vi "Teleop.vi"(10 "Match Info":T2={"Autonomous Elapsed Seconds"=0.0, "TeleOp Elapsed Seconds"=0.0, "Disabled Elapsed Seconds"=0.0, "Visited Autonomous"=FALSE, "Visited TeleOp"=FALSE, "Visited Disabled"=FALSE, "Autonomous Settings"={"Autonomous Style"=enum."Independent", "VI Refnum"=refnum}}, 11 "Call Context":T3) -> ()   [LabVIEW 2017]
doc: "This VI is called for each TeleOp packet received from the DS where the robot is not disabled. It is often used to read from the joysticks and update I/O or to update setpoints for timed control loops. It should complete and return within 20 milliseconds or it may miss DS packets."
uses:
  <vilib>/Rock Robotics/WPI/DriverStation/WPI_DriverStationDerivedRobotMode.ctl
  <vilib>/Rock Robotics/WPI/DriverStation/WPI_DriverStationMatch Info.ctl
  Type Definitions/Teleop States.ctl
  Type Definitions/Joystick Axes.ctl
  Type Definitions/joystick Buttons.ctl
  <vilib>/Rock Robotics/WPI/ThirdParty/Phoenix-LabVIEW/Motor Controller/Controls/CTRE_Phoenix_MotorControl_ControlMode.ctl
  <vilib>/Rock Robotics/WPI/Utilities/WPI_GetSetVariantRefNum.vi
  <vilib>/Rock Robotics/Network Tables/NT Write Number.vi
panel:
  in  "Manual Control":bool
  in  "Right Slide":dbl(slide) min=-0.15 max=0.15 step=0.01 scale=-0.2..0.2 scale format="%.2f"
  in  "Left Slide":dbl(slide) min=-0.15 max=0.15 step=0.01 scale=-0.2..0.2 scale format="%.2f"
  in  "Teleop Analyctical Data":T1
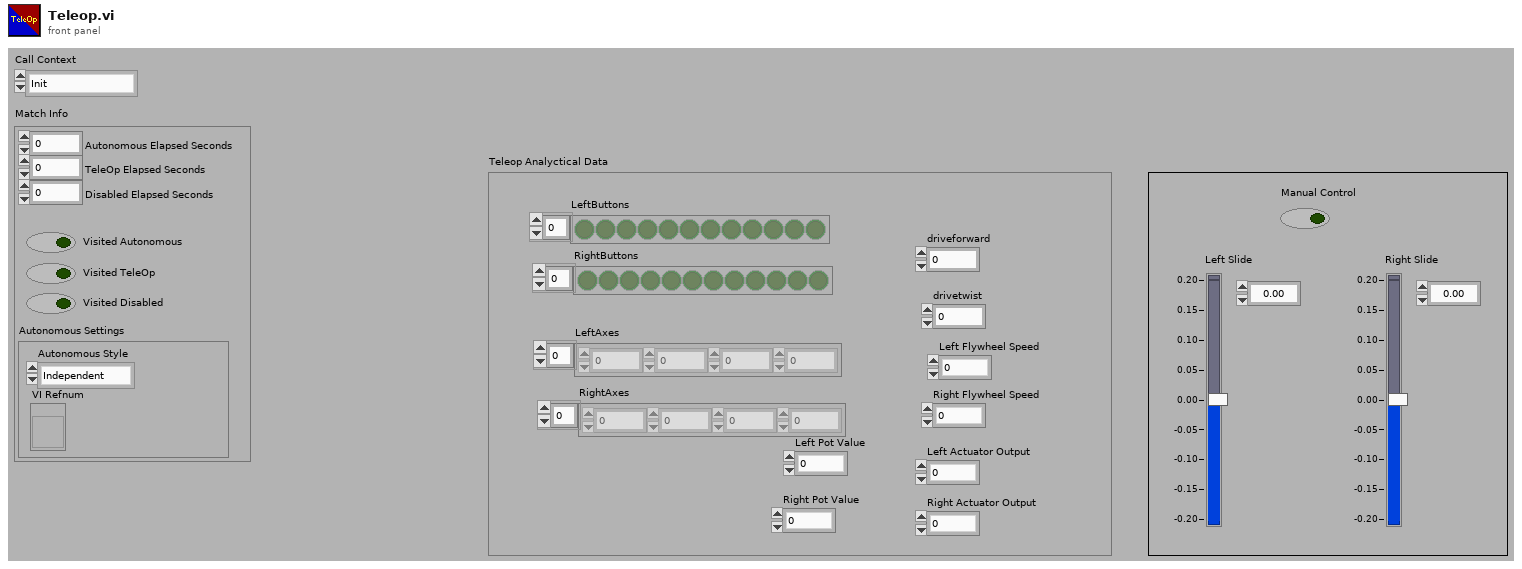
[diagram p1: front panel]
types:
  T1 = cluster{"LeftButtons":bool[], "RightButtons":bool[], "LeftAxes":dbl[], "RightAxes":dbl[], "driveforward":dbl, "drivetwist":dbl, "Left Flywheel Speed":dbl, "Right Flywheel Speed":dbl, "Left Actuator Output":dbl, "Right Actuator Output":dbl, "Left Pot Value":dbl, "Right Pot Value":dbl}
  T2 = typedef "WPI_DriverStationMatch Info.ctl" = cluster{"Autonomous Elapsed Seconds":dbl, "TeleOp Elapsed Seconds":dbl, "Disabled Elapsed Seconds":dbl, "Visited Autonomous":bool, "Visited TeleOp":bool, "Visited Disabled":bool, "Autonomous Settings":cluster{"Autonomous Style":enum16{"Iterative", "Independent"}, "VI Refnum":refnum<vi>}}
  T3 = typedef "WPI_DriverStationDerivedRobotMode.ctl" = enum16{"Init", "Execute", "Stop"}
  T4 = typedef "Teleop States.ctl" = enum16{"Start", "i_leftJoystick", "i_RightJoystick", "i_pot", "c_drive", "c_actuator", "c_flywheels", "output", "output actuator", "End"}
  T5 = typedef "Joystick Axes.ctl" = enum16{"X Axis", "Y Axis", "Twist", "Throttle"}
  T6 = typedef "joystick Buttons.ctl" = enum16{"Trigger", "Thumb", "buttom2", "buttom3", "button4", "button5", "button6"}
  T7 = typedef "WPI_JoystickDevRef.ctl" = cluster{"Device":T8}
  T8 = typedef "WPI_JoystickDeviceEnum.ctl" = enum16{"USB 0", "USB 1", "USB 2", "USB 3", "USB 4", "USB 5"}
  T9 = typedef "WPI_PotentiometerDevRef.ctl" = cluster{"DevStatus":errorcluster, "Analog Channel":T10, "Invert Output":bool}
  T10 = typedef "FPGA_AIChannel.ctl" = enum8{"AI 0", "AI 1", "AI 2", "AI 3", "AI MXP 0", "AI MXP 1", "AI MXP 2", "AI MXP 3", "Invalid"}
  T11 = typedef "CTRE_Phoenix_MotorControl_ControlMode.ctl" = u16
  T12 = typedef "WPI_RobotDriveDevRef.ctl" = cluster{"DevStatus":errorcluster, "Motors[]":T13[], "Square Inputs":bool, "Max Output":dbl}
  T13 = typedef "WPI_MotorControlDeviceRef.ctl" = cluster{"DeviceStatus":errorcluster, "Type":T14, "PWM":cluster{"PWM Channel":T15, "DeadBand":T16}, "CAN":cluster{"Device Number":u8, "SetOutput VI Ref":variant, "GetOutput VI Ref":variant, "Enable VI Ref":variant, "Disable VI Ref":variant, "Data":variant}, "Invert":bool, "DIO PWM":cluster{"PWM \"Enable\" Channel":T15, "DIOChannel":T17, "PWM Rate":dbl}}
  T14 = typedef "WPI_MotorControlType.ctl" = enum16{"PWM", "CAN", "DIO PWM"}
  T15 = typedef "FPGA_DIOPWMChannel.ctl" = enum8{"PWM 0", "PWM 1", "PWM 2", "PWM 3", "PWM 4", "PWM 5", "PWM 6", "PWM 7", "PWM 8", "PWM 9", "PWM MXP 0", "PWM MXP 1", "PWM MXP 2", "PWM MXP 3", "PWM MXP 4", "PWM MXP 5", "PWM MXP 6", "PWM MXP 7", "PWM MXP 8", "PWM MXP 9", "Invalid"}
  T16 = typedef "WPI_PWMDeadband.ctl" = cluster{"Name":string, "maxPositivePwm":i32, "minPositivePwm":i32, "centerPwm":i32, "maxNegativePwm":i32, "minNegativePwm":i32, "angularRange":u16}
  T17 = typedef "FPGA_DIOChannel.ctl" = enum8{"DIO 0", "DIO 1", "DIO 2", "DIO 3", "DIO 4", "DIO 5", "DIO 6", "DIO 7", "DIO 8", "DIO 9", "DIO MXP 0", "DIO MXP 1", "DIO MXP 2", "DIO MXP 3", "DIO MXP 4", "DIO MXP 5", "DIO MXP 6", "DIO MXP 7", "DIO MXP 8", "DIO MXP 9", "DIO MXP 10", "DIO MXP 11", "DIO MXP 12", "DIO MXP 13", "DIO MXP 14", "DIO MXP 15", "SPI Port CS1", "SPI Port CS2", "SPI Port CS3", "SPI Port MISO", "SPI Port MOSI", "Invalid"}
  T18 = typedef "WPI_ServoDeviceRef.ctl" = cluster{"DeviceStatus":errorcluster, "PWM Channel":T15, "DeadBand":T16}
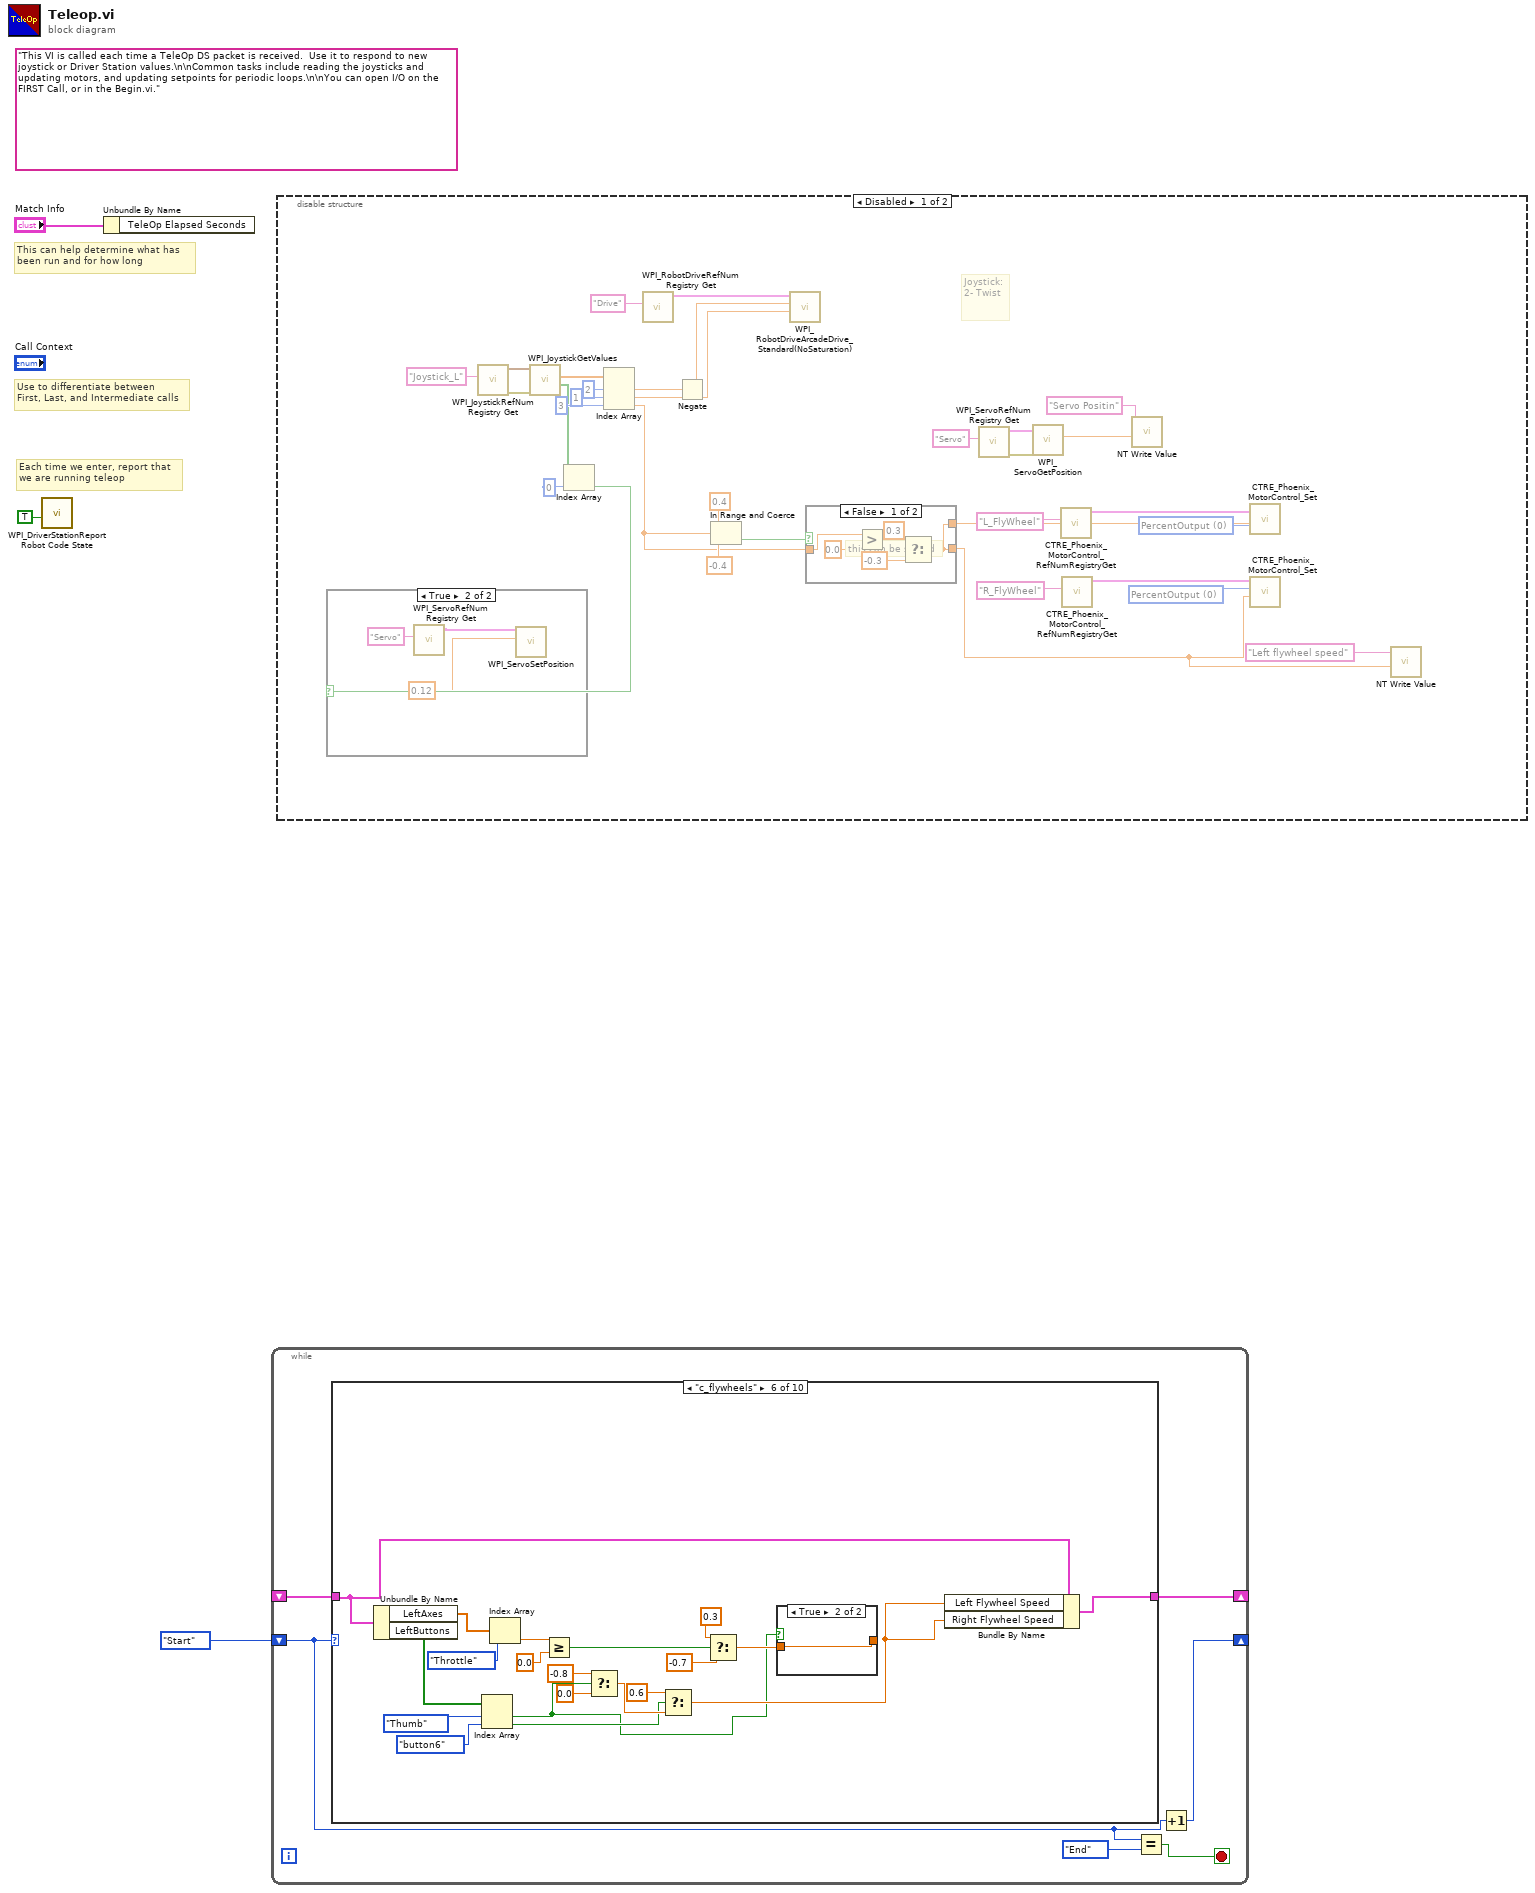
[diagram p0: block diagram]
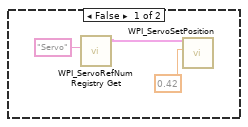
[diagram p2: hidden frame]
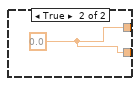
[diagram p3: hidden frame]
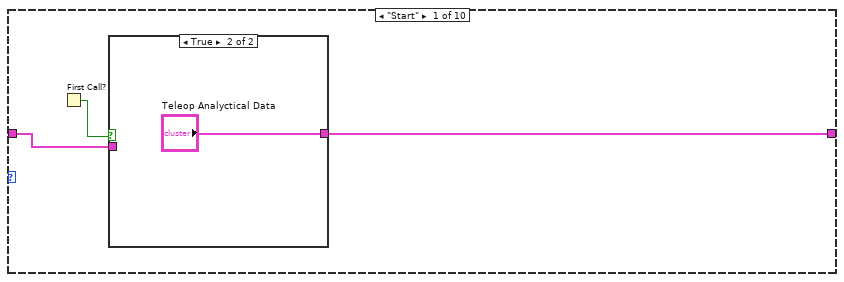
[diagram p5: hidden frame]
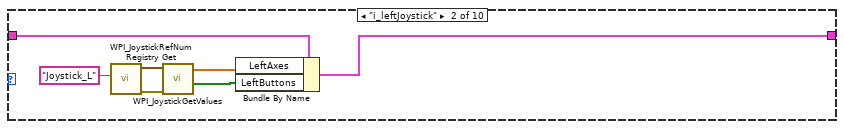
[diagram p7: hidden frame]
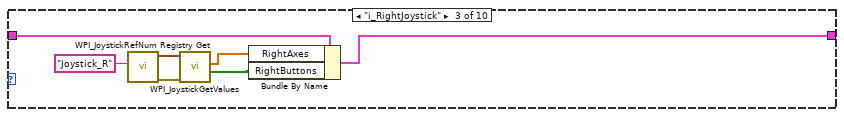
[diagram p8: hidden frame]
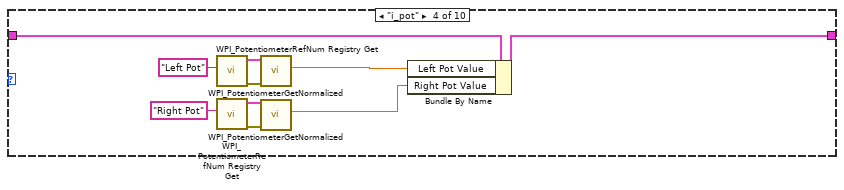
[diagram p9: hidden frame]
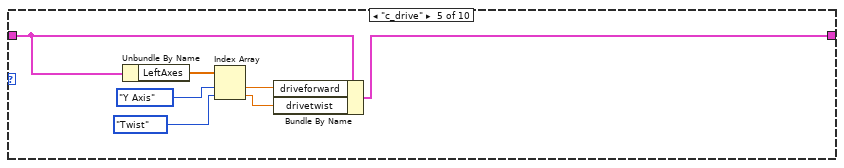
[diagram p10: hidden frame]
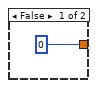
[diagram p11: hidden frame]
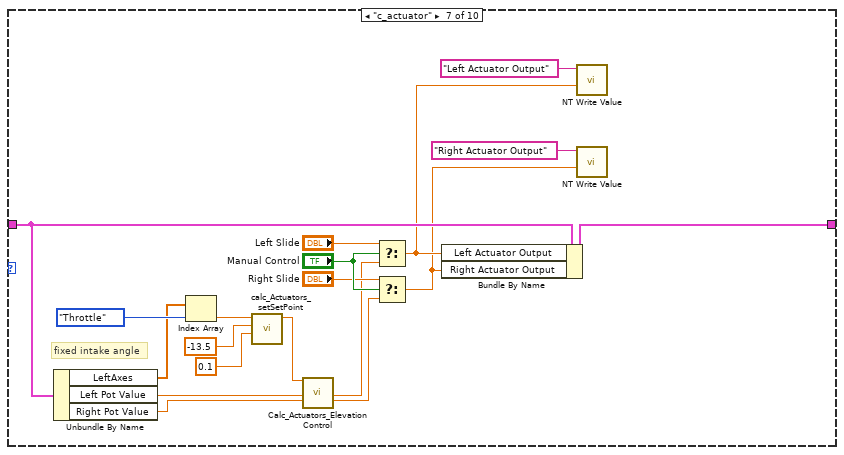
[diagram p12: hidden frame]
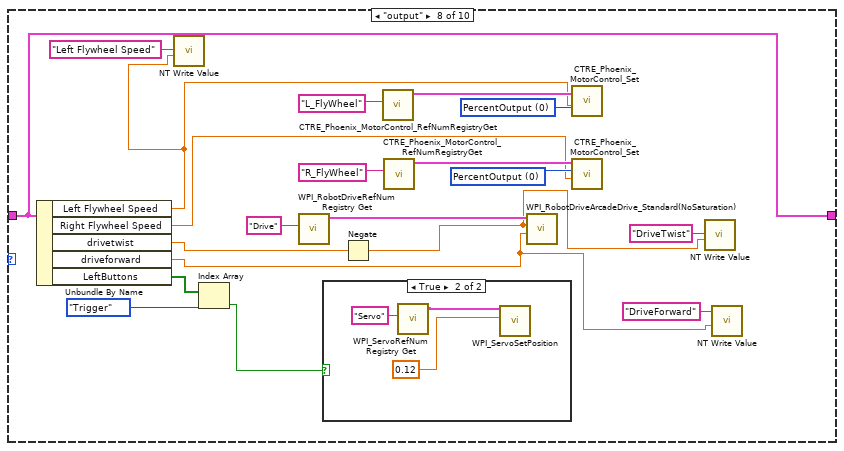
[diagram p13: hidden frame]
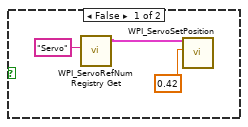
[diagram p14: hidden frame]
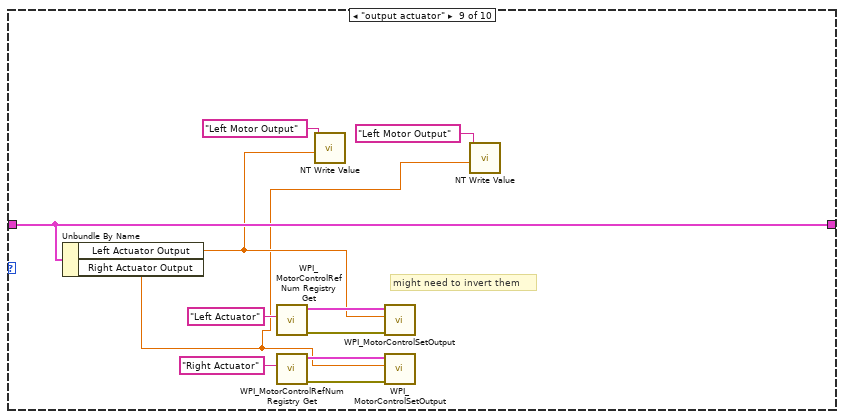
[diagram p15: hidden frame]
diagram:
  (unwired) "This VI is called each time a TeleOp DS packet is received.  Use it to respond to new joystick or Driver Station values.\n\nCommon tasks include reading the joysticks and updating motors, and updating setpoints for periodic loops.\n\nYou can open I/O on the FIRST Call, or in the Begin.vi."
  # "Each time we enter, report that\nwe are running teleop"
  # "Use to differentiate between\nFirst, Last, and Intermediate calls"
  # "This can help determine what has\nbeen run and for how long"
  n1 = call <vilib>:"WPI_DriverStationReport Robot Code State.vi"("TeleOp"=TRUE ("Autonomous")) -> ()  [unwired: 10 in, 1 out]
  n2 = Unbundle By Name("Match Info") -> ()  [unwired: 1 out]
  n3 = while {
    shift-right: [w8] -> _
    shift-left: _ -> [w9]
    shift-right: [w7] -> _
    shift-left: Teleop_States."Start" -> [w6]
    stop <- w4 stop-if-true
    n4 = case shown="\"c_flywheels\"" w6 {
      tunnel: w9 -> [w10 w17 w23 w32 w43 w57 w84 w106 w117 w124]
      tunnel: [w12 w16 w22 w29 w41 w56 w75 w106 w117 w124] -> w8
      frame "Start" {
        n5 = First Call?() -> (First Call?: T/F=w11:bool)
        n6 = case shown="True" w11 {
          tunnel: [w13 "Teleop Analyctical Data"] -> w12
          tunnel: w10 -> [w13 _]
          frame False {
          }
          frame True {
          }
        }
      }
      frame "i_leftJoystick" {
        n7 = call <vilib>:"WPI_JoystickRefNum Registry Get.vi"("refnum name"="Joystick_L") -> ("error out"=w20:errorcluster, "JoystickDevRef"=w21:T7)  [unwired: 9 in]
        n8 = call <vilib>:"WPI_JoystickGetValues.vi"("error in (no error)"=w20, "JoystickDevRef"=w21) -> ("Buttons"=w18:bool[], "Axes"=w15:dbl[])  [unwired: 5 in, 3 out]
        n9 = Bundle By Name(cluster=w17, "LeftAxes"=w15, "LeftButtons"=w18) -> (w16:T1)
      }
      frame "i_RightJoystick" {
        n10 = call <vilib>:"WPI_JoystickRefNum Registry Get.vi"("refnum name"="Joystick_R") -> ("error out"=w27:errorcluster, "JoystickDevRef"=w28:T7)  [unwired: 9 in]
        n11 = call <vilib>:"WPI_JoystickGetValues.vi"("error in (no error)"=w27, "JoystickDevRef"=w28) -> ("Buttons"=w25:bool[], "Axes"=w24:dbl[])  [unwired: 5 in, 3 out]
        n12 = Bundle By Name(cluster=w23, "RightAxes"=w24, "RightButtons"=w25) -> (w22:T1)
      }
      frame "i_pot" {
        n13 = call <vilib>:"WPI_PotentiometerRefNum Registry Get.vi"("refnum name"="Left Pot") -> ("error out"=w35:errorcluster, "PotDevRef"=w36:T9)  [unwired: 9 in]
        n14 = call <vilib>:"WPI_PotentiometerRefNum Registry Get.vi"("refnum name"="Right Pot") -> ("error out"=w38:errorcluster, "PotDevRef"=w37:T9)  [unwired: 9 in]
        n15 = call <vilib>:"WPI_PotentiometerGetNormalized.vi"("error in"=w35, "PotDevRef"=w36) -> ("Normalized Value"=w31:dbl)  [unwired: 7 in, 2 out]
        n16 = call <vilib>:"WPI_PotentiometerGetNormalized.vi"("error in"=w38, "PotDevRef"=w37) -> ("Normalized Value"=w30:dbl)  [unwired: 7 in, 2 out]
        n17 = Bundle By Name(cluster=w32, "Left Pot Value"=w31, "Right Pot Value"=w30) -> (w29:T1)
      }
      frame "c_drive" {
        n18 = Unbundle By Name(w43) -> ("LeftAxes"=w44:dbl[])
        n19 = Index Array(array=w44, index #1=Joystick_Axes."Y Axis", index #2=Joystick_Axes."Twist") -> (element #1=w42:dbl, element #2=w40:dbl)
        n20 = Bundle By Name(cluster=w43, "driveforward"=w42, "drivetwist"=w40) -> (w41:T1)
      }
      frame "c_flywheels" {
        n21 = Unbundle By Name(w57) -> ("LeftAxes"=w65:dbl[], "LeftButtons"=w64:bool[])
        n22 = Index Array(array=w64, index #1=joystick_Buttons."Thumb" ("Enum"), index #2=joystick_Buttons."button6" ("Enum")) -> (element #1=w46:bool, element #2=w47:bool)
        n23 = Index Array(array=w65, index=Joystick_Axes."Throttle" ("Enum")) -> (element=w49:dbl)
        n24 = Greater Or Equal?(x=w49, y=0.0) -> (x >= y?=w48:bool)
        n25 = Select(t=-0.8, s=w46, f=0.0) -> (s? t:f=w52:dbl)
        n26 = Select(t=0.6, s=w47, f=w52) -> (s? t:f=w50:dbl)
        n27 = Select(t=0.3, s=w48, f=-0.7) -> (s? t:f=w58:dbl)
        n28 = case shown="True" w46 {
          tunnel: [0 w67] -> _
          tunnel: w58 -> [_ w67]
          frame False {
          }
          frame True {
          }
        }
        n29 = Bundle By Name(cluster=w57, "Left Flywheel Speed"=w50, "Right Flywheel Speed"=w50) -> (w56:T1)
      }
      frame "c_actuator" {
        # "fixed intake angle"
        n30 = Unbundle By Name(w84) -> ("LeftAxes"=w80:dbl[], "Left Pot Value"=w83:dbl, "Right Pot Value"=w82:dbl)
        n31 = Index Array(array=w80, index=Joystick_Axes."Throttle" ("Enum")) -> (element=w79:dbl)
        n32 = call "calc_Actuators_setSetPoint.vi"("Throttle Deadband (0.1)"=0.1, "Fixed Intake Angle"=-13.5, "Joystick Axis Value"=w79) -> ("Angle Setpoint"=w76:dbl)  [unwired: 7 in]
        n33 = call "Calc_Actuators_Elevation Control.vi"("Elev_Setpoint"=w76, "Vpot_Left"=w83, "Vpot_Right"=w82) -> ("Power_Left"=w71:dbl, "Power_Right"=w70:dbl)  [unwired: 15 in]
        n34 = Select(t="Left Slide", s="Manual Control", f=w71) -> (s? t:f=w69:dbl)
        n35 = Select(t="Right Slide", s="Manual Control", f=w70) -> (s? t:f=w68:dbl)
        n36 = Bundle By Name(cluster=w84, "Left Actuator Output"=w69, "Right Actuator Output"=w68) -> (w75:T1)
        n37 = call-poly <vilib>:"NT Write Value.vi"("Numeric"=w69, "Name"="Left Actuator Output") -> ()  [unwired: 9 in, 1 out]
        n38 = call-poly <vilib>:"NT Write Value.vi"("Numeric"=w68, "Name"="Right Actuator Output") -> ()  [unwired: 9 in, 1 out]
      }
      frame "output" {
        w100 = T11 0 items=["PercentOutput"=0, "Position"=1, "Velocity"=2, "Current"=3, "Follower"=5, "MotionProfile"=6, "MotionMagic"=7, "MotionMagicArc"=8, "MotionProfileArc"=10, "Disabled"=15] ("Control Mode")
        w101 = T11 0 items=["PercentOutput"=0, "Position"=1, "Velocity"=2, "Current"=3, "Follower"=5, "MotionProfile"=6, "MotionMagic"=7, "MotionMagicArc"=8, "MotionProfileArc"=10, "Disabled"=15] ("Control Mode")
        n39 = Unbundle By Name(w106) -> ("Left Flywheel Speed"=w91:dbl, "Right Flywheel Speed"=w99:dbl, "drivetwist"=w96:dbl, "driveforward"=w87:dbl, "LeftButtons"=w95:bool[])
        n40 = call-poly <vilib>:"NT Write Value.vi"("Numeric"=w91, "Name"="Left Flywheel Speed") -> ()  [unwired: 9 in, 1 out]
        n41 = Index Array(array=w95, index=joystick_Buttons."Trigger" ("Enum")) -> (element=w93:bool)
        n42 = call <vilib>:"WPI_RobotDriveRefNum Registry Get.vi"("refnum name"="Drive") -> ("RobotDriveDevRef"=w97:T12)  [unwired: 9 in, 1 out]
        n43 = case shown="True" w93 {
          frame False {
            n44 = call <vilib>:"WPI_ServoRefNum Registry Get.vi"("refnum name"="Servo") -> ("ServoDeviceRef"=w108:T18)  [unwired: 9 in, 1 out]
            n45 = call <vilib>:"WPI_ServoSetPosition.vi"("Position"=0.42, "ServoDeviceRef"=w108) -> ()  [unwired: 8 in, 2 out]
          }
          frame True {
            n46 = call <vilib>:"WPI_ServoRefNum Registry Get.vi"("refnum name"="Servo") -> ("ServoDeviceRef"=w112:T18)  [unwired: 9 in, 1 out]
            n47 = call <vilib>:"WPI_ServoSetPosition.vi"("Position"=0.12, "ServoDeviceRef"=w112) -> ()  [unwired: 8 in, 2 out]
          }
        }
        n48 = Negate(x=w96) -> (-x=w88:dbl)
        n49 = call <vilib>:"CTRE_Phoenix_MotorControl_RefNumRegistryGet.vi"("refnum name"="L_FlyWheel") -> ("PhoenixMotorControlDevRef"=w103:T13)  [unwired: 9 in, 1 out]
        n50 = call <vilib>:"CTRE_Phoenix_MotorControl_RefNumRegistryGet.vi"("refnum name"="R_FlyWheel") -> ("PhoenixMotorControlDevRef"=w102:T13)  [unwired: 9 in, 1 out]
        n51 = call <vilib>:"WPI_RobotDriveArcadeDrive_Standard(NoSaturation).vi"("Y axis value"=w87, "X axis value"=w88, "RobotDriveDevRef"=w97) -> ()  [unwired: 1 in, 8 out]
        n52 = call <vilib>:"CTRE_Phoenix_MotorControl_Set.vi"("Output"=w91, "Control Mode"=w101, "PhoenixMotorControlDevRef"=w103) -> ()  [unwired: 7 in, 2 out]
        n53 = call <vilib>:"CTRE_Phoenix_MotorControl_Set.vi"("Output"=w99, "Control Mode"=w100, "PhoenixMotorControlDevRef"=w102) -> ()  [unwired: 7 in, 2 out]
        n54 = call-poly <vilib>:"NT Write Value.vi"("Numeric"=w88, "Name"="DriveTwist") -> ()  [unwired: 9 in, 1 out]
        n55 = call-poly <vilib>:"NT Write Value.vi"("Numeric"=w87, "Name"="DriveForward") -> ()  [unwired: 9 in, 1 out]
      }
      frame "output actuator" {
        # "might need to invert them"
        n56 = Unbundle By Name(w117) -> ("Left Actuator Output"=w116:dbl, "Right Actuator Output"=w115:dbl)
        n57 = call <vilib>:"WPI_MotorControlRefNum Registry Get.vi"("refnum name"="Left Actuator") -> ("error out"=w121:errorcluster, "MotorControlDevRef"=w123:T13)  [unwired: 9 in]
        n58 = call <vilib>:"WPI_MotorControlRefNum Registry Get.vi"("refnum name"="Right Actuator") -> ("error out"=w118:errorcluster, "MotorControlDevRef"=w120:T13)  [unwired: 9 in]
        n59 = call-poly <vilib>:"NT Write Value.vi"("Numeric"=w116, "Name"="Left Motor Output") -> ()  [unwired: 9 in, 1 out]
        n60 = call <vilib>:"WPI_MotorControlSetOutput.vi"("error in (no error)"=w121, "Output"=w116, "MotorControlDevRef"=w123) -> ()  [unwired: 6 in, 3 out]
        n61 = call <vilib>:"WPI_MotorControlSetOutput.vi"("error in (no error)"=w118, "Output"=w115, "MotorControlDevRef"=w120) -> ()  [unwired: 6 in, 3 out]
        n62 = call-poly <vilib>:"NT Write Value.vi"("Numeric"=w115, "Name"="Left Motor Output") -> ()  [unwired: 9 in, 1 out]
      }
      frame "End" {
      }
    }
    n63 = Equal?(x=w6, y=Teleop_States."End" ("States")) -> (x = y?=w4:bool)
    n64 = Increment(x=w6) -> (x+1=w7:T4)
  }
  n65 = disable-structure shown="Disabled" {
    frame Disabled {
      w138 = T11 0 items=["PercentOutput"=0, "Position"=1, "Velocity"=2, "Current"=3, "Follower"=5, "MotionProfile"=6, "MotionMagic"=7, "MotionMagicArc"=8, "MotionProfileArc"=10, "Disabled"=15] ("Control Mode")
      w139 = T11 0 items=["PercentOutput"=0, "Position"=1, "Velocity"=2, "Current"=3, "Follower"=5, "MotionProfile"=6, "MotionMagic"=7, "MotionMagicArc"=8, "MotionProfileArc"=10, "Disabled"=15] ("Control Mode")
      # "Joystick:\n2- Twist"
      # "this can be scaled"
      n66 = call <vilib>:"WPI_JoystickRefNum Registry Get.vi"("refnum name"="Joystick_L") -> ("error out"=w156:errorcluster, "JoystickDevRef"=w155:T7)  [unwired: 9 in]
      n67 = call <vilib>:"WPI_JoystickGetValues.vi"("error in (no error)"=w156, "JoystickDevRef"=w155) -> ("Buttons"=w132:bool[], "Axes"=w154:dbl[])  [unwired: 5 in, 3 out]
      n68 = Index Array(array=w132, index=0) -> (element=w130:bool)
      n69 = case shown="True" w130 {
        frame False {
          n70 = call <vilib>:"WPI_ServoRefNum Registry Get.vi"("refnum name"="Servo") -> ("ServoDeviceRef"=w159:T18)  [unwired: 9 in, 1 out]
          n71 = call <vilib>:"WPI_ServoSetPosition.vi"("Position"=0.42, "ServoDeviceRef"=w159) -> ()  [unwired: 8 in, 2 out]
        }
        frame True {
          n72 = call <vilib>:"WPI_ServoRefNum Registry Get.vi"("refnum name"="Servo") -> ("ServoDeviceRef"=w163:T18)  [unwired: 9 in, 1 out]
          n73 = call <vilib>:"WPI_ServoSetPosition.vi"("Position"=0.12, "ServoDeviceRef"=w163) -> ()  [unwired: 8 in, 2 out]
        }
      }
      n74 = Index Array(array=w154, index #1=2 ("index"), index #2=1 ("index"), index #3=3 ("index")) -> (element #1=w148:dbl, element #2=w149:dbl, element #3=w135:dbl)
      n75 = call <vilib>:"WPI_RobotDriveRefNum Registry Get.vi"("refnum name"="Drive") -> ("RobotDriveDevRef"=w152:T12)  [unwired: 9 in, 1 out]
      n76 = Negate(x=w148) -> (-x=w147:dbl)
      n77 = In Range and Coerce(upper limit=0.4, x=w135, lower limit=-0.4) -> (In Range?=w137:bool)  [unwired: 1 out]
      n78 = call <vilib>:"WPI_RobotDriveArcadeDrive_Standard(NoSaturation).vi"("Y axis value"=w149, "X axis value"=w147, "RobotDriveDevRef"=w152) -> ()  [unwired: 1 in, 8 out]
      n79 = case shown="False" w137 {
        tunnel: [w164 w170] -> w136
        tunnel: w135 -> [w168 _]
        tunnel: [w164 w170] -> w133
        frame False {
          n80 = Greater?(x=w168, y=0.0) -> (0:w167:bool)
          n81 = Select(t=0.3, s=w167, f=-0.3) -> (s? t:f=w164:dbl)
        }
        frame True {
          w170 = 0.0 ("upper limit")
        }
      }
      n82 = call <vilib>:"WPI_ServoRefNum Registry Get.vi"("refnum name"="Servo") -> ("error out"=w128:errorcluster, "ServoDeviceRef"=w127:T18)  [unwired: 9 in]
      n83 = call <vilib>:"WPI_ServoGetPosition.vi"("error in (no error)"=w128, "ServoDeviceRef"=w127) -> ("Position"=w126:dbl)  [unwired: 7 in, 2 out]
      n84 = call <vilib>:"CTRE_Phoenix_MotorControl_RefNumRegistryGet.vi"("refnum name"="L_FlyWheel") -> ("PhoenixMotorControlDevRef"=w141:T13)  [unwired: 9 in, 1 out]
      n85 = call <vilib>:"CTRE_Phoenix_MotorControl_RefNumRegistryGet.vi"("refnum name"="R_FlyWheel") -> ("PhoenixMotorControlDevRef"=w140:T13)  [unwired: 9 in, 1 out]
      n86 = call-poly <vilib>:"NT Write Value.vi"("Numeric"=w126, "Name"="Servo Positin") -> ()  [unwired: 9 in, 1 out]
      n87 = call <vilib>:"CTRE_Phoenix_MotorControl_Set.vi"("Output"=w136, "Control Mode"=w139, "PhoenixMotorControlDevRef"=w141) -> ()  [unwired: 7 in, 2 out]
      n88 = call <vilib>:"CTRE_Phoenix_MotorControl_Set.vi"("Output"=w133, "Control Mode"=w138, "PhoenixMotorControlDevRef"=w140) -> ()  [unwired: 7 in, 2 out]
      n89 = call-poly <vilib>:"NT Write Value.vi"("Numeric"=w133, "Name"="Left flywheel speed") -> ()  [unwired: 9 in, 1 out]
    }
    frame Enabled {
    }
  }
